vi "Tetra_TxReg_48.vi"(0 "COMPORT":refnum<visa-resource-name>="COM4", 7 "error in (no error)":errorcluster, 8 "Open Ser(t)":bool, 9 "R(t)":bool, 12 "Close Ser(t)":bool, 13 "BPF":bool, 15 "NOTCH":bool, 17 "ATTN_SPI":u32 max=31 step=1) -> (14 "bpf":bool, 16 "notch":bool, 18 "attn_spi":u8, 20 "comport":refnum<visa-resource-name>="COM4", 27 "error out":errorcluster)   [LabVIEW 2018]
panel:
  out "output 2":string
  out "reserved":bool
  out "input":string
  in  "RESERVED":bool
  # "readback"
  # "Input"
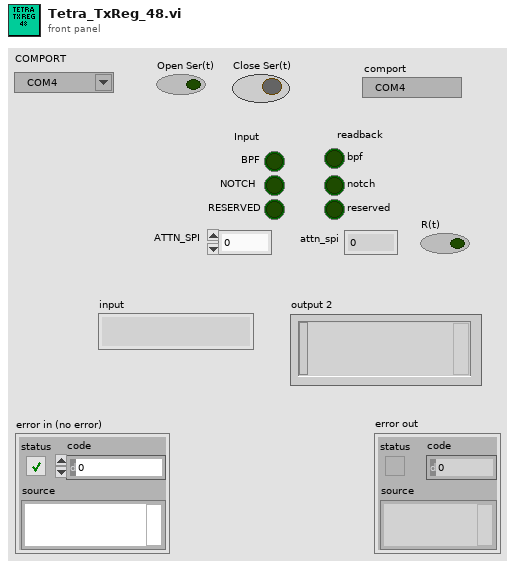
[diagram p1: front panel]
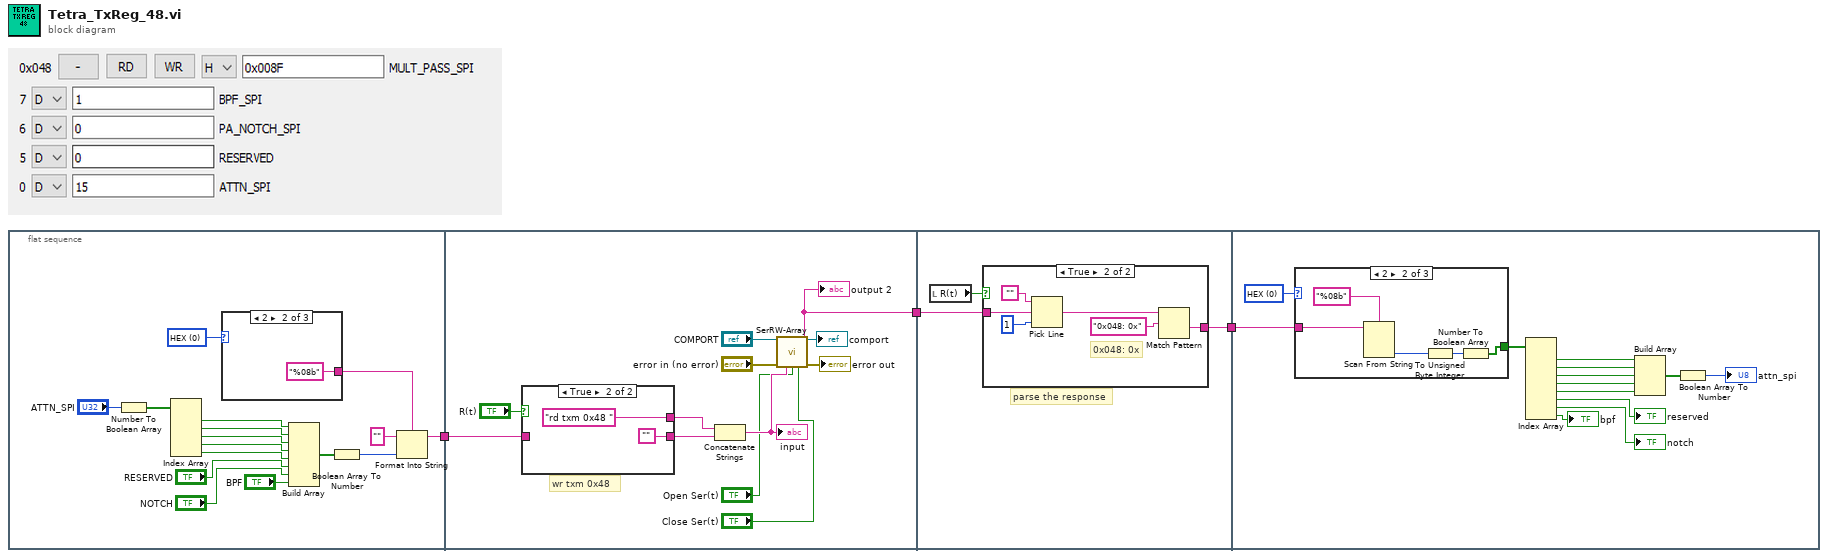
[diagram p0: block diagram]
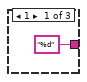
[diagram p2: hidden frame]
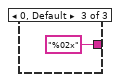
[diagram p3: hidden frame]
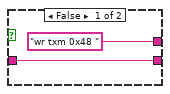
[diagram p4: hidden frame]
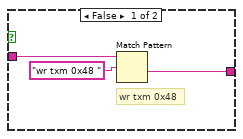
[diagram p5: hidden frame]
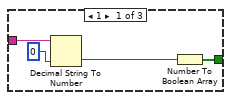
[diagram p6: hidden frame]
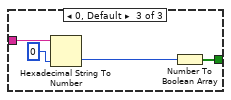
[diagram p7: hidden frame]
diagram:
  n1 = flat-sequence {
    tunnel: [w4] -> w3
    tunnel: w3 -> [w32]
    tunnel: [w27] -> w2
    tunnel: w2 -> [w41]
    tunnel: [w39] -> w1
    tunnel: w1 -> [w52]
    frame #0 {
      w19 = u16 0 items=["HEX", "DEC", "BIN"] ("Outp Form")
      n2 = Number To Boolean Array(number="ATTN_SPI") -> (Boolean array=w11:bool[])
      n3 = Index Array(array=w11) -> (element #1=w12:bool, element #2=w13:bool, element #3=w14:bool, element #4=w15:bool, element #5=w16:bool)  [unwired: 5 in]
      n4 = case shown="2" w19 {
        tunnel: ["%d" ("format string") "%08b" ("format string") "%02x" ("format string")] -> w18
        frame 1 {
        }
        frame 2 {
        }
        frame 0, Default {
        }
      }
      n5 = Build Array(w12, w13, w14, w15, w16, "RESERVED", "NOTCH", "BPF") -> (w10:bool[])
      n6 = Boolean Array To Number(Boolean array=w10) -> (number=w17:u32)
      n7 = Format Into String(format string=w18, initial string="", w17) -> (resulting string=w4:string)  [unwired: 1 in, 1 out]
    }
    frame #1 {
      # "wr txm 0x48"
      n8 = case shown="True" "R(t)" {
        tunnel: w32 -> [w36 _]
        tunnel: [w36 ""] -> w31
        tunnel: ["wr txm 0x48 " "rd txm 0x48 "] -> w30
        frame False {
        }
        frame True {
        }
      }
      n9 = Concatenate Strings(w30, w31) -> (w26:string)
      "input" <- w26
      n10 = call "SerRW-Array.vi"("COMPORT"="COMPORT", "error in (no error)"="error in (no error)", "Command ( ; seperation)"=w26, "Open Serial"="Open Ser(t)", "Close Serial"="Close Ser(t)") -> ("comport"=→"comport":refnum<visa-resource-name>, "string"=w27:string, "error out"=→"error out":errorcluster)  [unwired: 4 in, 4 out]
      "output 2" <- w27
    }
    frame #2 {
      # "parse the response"
      n11 = local read "R(t)"() -> (w40:bool)
      n12 = case shown="True" w40 {
        tunnel: w41 -> [w44 w49]
        tunnel: [w42 w45] -> w39
        frame False {
          # "wr txm 0x48"
          n13 = Match Pattern(string=w44, regular expression="wr txm 0x48 ") -> (after substring=w42:string)  [unwired: 1 in, 3 out]
        }
        frame True {
          # "0x048: 0x"
          n14 = Pick Line(string ("")="", multi-line string=w49, line index=1) -> (output string=w47:string)
          n15 = Match Pattern(string=w47, regular expression="0x048: 0x") -> (after substring=w45:string)  [unwired: 1 in, 3 out]
        }
      }
    }
    frame #3 {
      w51 = u16 0 items=["HEX", "DEC", "BIN"] ("Outp Form")
      n16 = case shown="2" w51 {
        tunnel: w52 -> [w67 w72 w74]
        tunnel: [w65 w70 w75] -> w57
        frame 1 {
          n17 = Decimal String To Number(string=w67, default (0L)=u16 0 ("default (0 I32)")) -> (number=w64:u16)  [unwired: 1 in, 1 out]
          n18 = Number To Boolean Array(number=w64) -> (Boolean array=w65:bool[])
        }
        frame 2 {
          n19 = Scan From String(format string="%08b", input string=w72) -> (output 1=w69:i32)  [unwired: 3 in, 3 out]
          n20 = To Unsigned Byte Integer(number=w69) -> (unsigned 8bit integer=w68:u8)
          n21 = Number To Boolean Array(number=w68) -> (Boolean array=w70:bool[])
        }
        frame 0, Default {
          n22 = Hexadecimal String To Number(string=w74, default (0uL)=u8 0 ("default (0 U32)")) -> (number=w76:u8)  [unwired: 1 in, 1 out]
          n23 = Number To Boolean Array(number=w76) -> (Boolean array=w75:bool[])
        }
      }
      n24 = Index Array(array=w57) -> (element #1=w58:bool, element #2=w59:bool, element #3=w60:bool, element #4=w61:bool, element #5=w62:bool, element #6=→"reserved":bool, element #7=→"notch":bool, element #8=→"bpf":bool)  [unwired: 8 in]
      n25 = Build Array(w58, w59, w60, w61, w62) -> (w63:bool[])
      n26 = Boolean Array To Number(Boolean array=w63) -> (number=→"attn_spi":u32)
    }
  }
